vi "GetDataFiles.vi"(4 "Color scheme":string, 6 "Settings":T1={"Name of test"="", "Date"=timestamp(0 s since 1904-01-01), "Location"="", "Template"="", "Soundcard"="", "resolution"=32, "Sampling rate"=48000, "Ch1 Gain "=25.0, "Ch2 Gain"=10.0, "Sample time (s)"=0.3, "Pre-trigger (s)"=0.01, "Hammer Threshold"=10.0, "Positions"=12, "Taps/Position"=5, "Set Names"="", "Freq resolution"=10.0, "Hammer cutoff"=0.0, "Mic cutoff"=0.0, "Double bounce "=0.0, "Hammer Cal"=10.0, "dB Offset"=0.0, "Accel Cal"=10.0, "Vibrometer Cal"=0.0, "Mic Cal"=0.0, "Output"=2, "Voltage Cal"=1.0, "Vibrometer Port"="ASRL27::INSTR", "Range"=4, "High Pass"=2, "Bandwidth"=4, "X Range"=[], "Y Range"=[], "dB Spread"=0.0, "Trigger"=0, "Ch_1"=25, "Ch_2"=25, "flip?"=FALSE, "60Hz"=FALSE, "Time offset"=0.0, "Piezo Cal"=1.0, "Default Notes"=""} {"Ch_2" min=1 step=1; "Ch_1" min=1 max=100 step=1; "Trigger" items=["Hammer (force)", "Self-tap", "Spacebar"]; "Bandwidth" items=["1 kHz"=1, "5 kHz"=5, "10 kHz"=10, "25 kHz"=25, "50 kHz"=50, "100 kHz"=100]; "High Pass" items=["Off", "13 Hz", "104 Hz"]; "Range" items=["10 mm/s"=1, "20 mm/s"=2, "50 mm/s"=5, "100 mm/s"=10, "200 mm/s"=20, "500 mm/s"=50, "1 m/s"=100, "2 m/s"=200]; "Output" items=["Accelerometer", "Speed (from acceleration)", "Microphone", "Vibrometer", "Piezo"]; "Voltage Cal" format="%#_13g"; "Ch2 Gain" format="%#_13g"; "Ch1 Gain" format="%#_13g"; "Double bounce" min=0.0; "Mic cutoff" min=0.0 format="%#_4g"; "Hammer cutoff" min=0.0 format="%#_4g"; "Freq resolution" min=0.0; "Pre-trigger (s)" format="%#_13g"; "Date" format="%<%H:%M\n%d/%m/%y>T"; "resolution" items=["16 bit"=16, "24 bit"=24, "32 bit"=32]; "Sampling rate" items=["22050 samp/s"=22050, "44100 samp/s"=44100, "48000 samp/s"=48000]}, 7 "View":u16(ring) items=["Raw", "Volts", "Units (Pa, N, etc)"], 8 "plots":refnum<vi>[](array[refnum]), 9 "Show history":bool, 10 "path":path, 11 "Method":enum16{"Sqrt(H1H2)", "H1", "H2"}(ring)) -> (0 "Microphone":cluster{dbl, "dt":dbl, "Y":dbl[]}[](graph), 1 "Average FRF":cluster{dbl, "df":dbl, dbl[]}[](graph), 2 "Last Data Set":waveform(dbl)[](array[waveform]), 3 "Hammer":cluster{dbl, "dt":dbl, "Y":dbl[]}[](graph), 5 "Hammer Spectra":cluster{dbl, "df":dbl, "FFT {X}":dbl[]}[](array[cluster]))   [LabVIEW 2022 SP3]
uses:
  PreferencesControl.ctl
  Mic/Mic_Global.vi
panel:
  out "Line":dbl
  out "Banner":string
  # "Hz"
  # "dB"
  # "dB"
  # "sec"
  # "sec"
  # "mV/Pa"
  # "mV/m/s2"
  # "mV/mm/s"
  # "V/N"
  # "sec"
  # "sec"
  # "mV/N"
  # "a.u."
  # "a.u."
  # "sec"
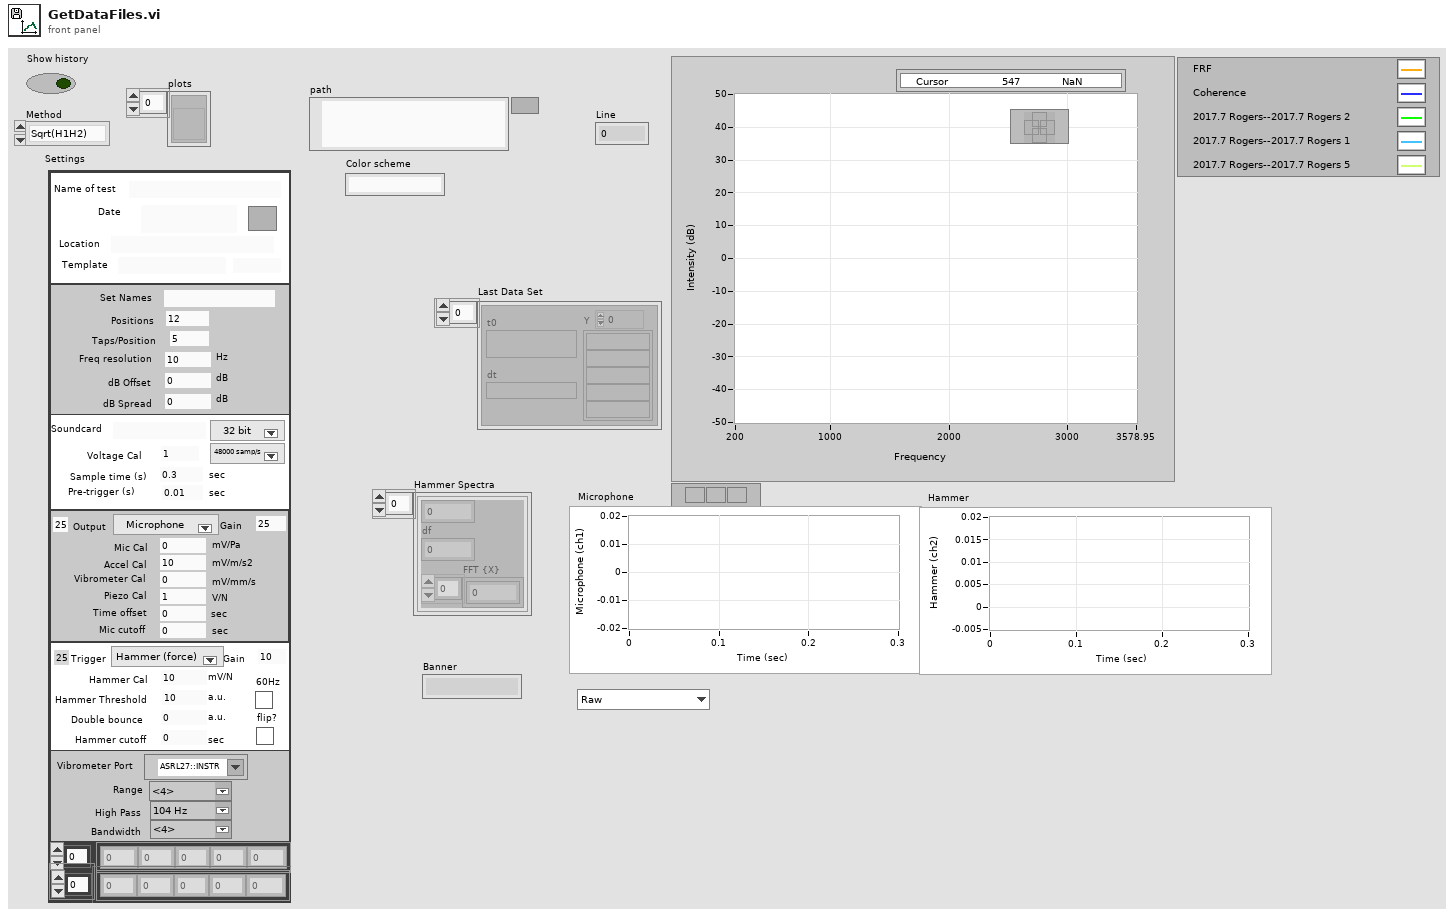
[diagram p1: front panel]
types:
  T1 = typedef "PreferencesControl.ctl" = cluster{"Name of test":string, "Date":timestamp, "Location":string, "Template":string, "Soundcard":string, "resolution":u16, "Sampling rate":u16, "Ch1 Gain ":dbl, "Ch2 Gain":dbl, "Sample time (s)":dbl, "Pre-trigger (s)":dbl, "Hammer Threshold":dbl, "Positions":i16, "Taps/Position":i16, "Set Names":string, "Freq resolution":dbl, "Hammer cutoff":dbl, "Mic cutoff":dbl, "Double bounce ":dbl, "Hammer Cal":dbl, "dB Offset":dbl, "Accel Cal":dbl, "Vibrometer Cal":dbl, "Mic Cal":dbl, "Output":u16, "Voltage Cal":dbl, "Vibrometer Port":refnum<visa-resource-name>, "Range":u16, "High Pass":u16, "Bandwidth":u16, "X Range":cluster{"Minimum":dbl, "Maximum":dbl, "Increment":dbl, "Minor Increment":dbl, "Start":dbl}[], "Y Range":cluster{"Minimum":dbl, "Maximum":dbl, "Increment":dbl, "Minor Increment":dbl, "Start":dbl}[], "dB Spread":dbl, "Trigger":u16, "Ch_1":u8, "Ch_2":u8, "flip?":bool, "60Hz":bool, "Time offset":dbl, "Piezo Cal":dbl, "Default Notes":string}
  T2 = cluster{"Hammer":cluster{dbl, "dt":dbl, "Y":dbl[]}[], "Microphone":cluster{dbl, "dt":dbl, "Y":dbl[]}[], "Hammer Spectrum":cluster{dbl, "dt":dbl, "Y":dbl[]}[], "FRF":cluster{dbl, "dt":dbl, "Y":dbl[]}[]}
  T3 = cluster{"Alerts":bool, "Log X Axis":bool, "dB scale":bool, "Averaging":bool, "Fade":dbl, "Centroids?":bool, "line thickness":u8}
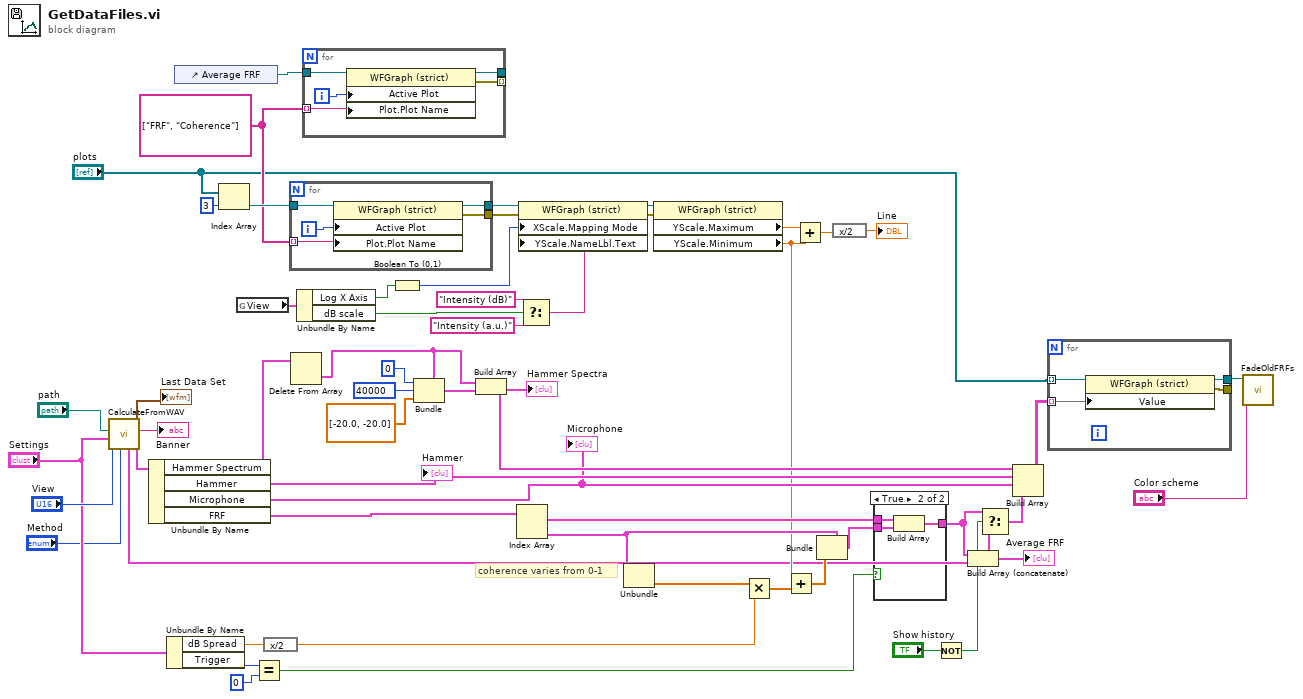
[diagram p0: block diagram]
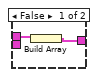
[diagram p2: hidden frame]
diagram:
  w40 = string[] ["FRF", "Coherence"]
  # "coherence varies from 0-1"
  n1 = call "CalculateFromWAV.vi"("Method"="Method", "View"="View", "Settings"="Settings", "path"="path") -> ("Plots"=w44:T2, "Alert"=→"Banner":string, "Last Data Set"=→"Last Data Set":waveform(dbl)[], "Old FRFs"=w10:cluster{dbl, "dt":dbl, "Y":dbl[]}[])  [unwired: 3 in, 1 out]
  n2 = Unbundle By Name(w44) -> ("Hammer Spectrum"=w43:cluster{dbl, "dt":dbl, "Y":dbl[]}[], "Hammer"=w34:cluster{dbl, "dt":dbl, "Y":dbl[]}[], "Microphone"=w33:cluster{dbl, "dt":dbl, "Y":dbl[]}[], "FRF"=w41:cluster{dbl, "dt":dbl, "Y":dbl[]}[])
  "Microphone" <- w33
  "Hammer" <- w34
  n3 = Unbundle By Name("Settings") -> ("dB Spread"=w13:dbl, "Trigger"=w27:u16)
  n4 = control-ref of="Average FRF"() -> (w48:refnum<vi>)
  n5 = Index Array(array="plots", index=3) -> (element=w51:refnum<vi>)
  n6 = global read "Mic_Global.vi" "View"() -> (w45:T3)
  n7 = Equal?(x=w27, y=u16 0 ("Input")) -> (x = y?=w26:bool)
  n8 = expression code="x/2"(w13) -> (w11:dbl)
  n9 = for {
    tunnel: w51 -> [w61]
    tunnel: w40 -> [w60] mode=indexing
    tunnel: [w59] -> w47
    tunnel: [w58] -> w30
    i -> [w62]
    n10 = property on="Property Node" class="WFGraph (strict)"(reference=w61, "Active Plot"=w62, "Plot.Plot Name"=w60) -> (reference out=w59:refnum<vi>, error out=w58:errorcluster)  [unwired: 1 in]
  }
  n11 = Delete From Array(array=w43) -> (deleted portion=w53:cluster{dbl, "dt":dbl, "Y":dbl[]})  [unwired: 2 in, 1 out]
  n12 = Unbundle By Name(w45) -> ("Log X Axis"=w25:bool, "dB scale"=w21:bool)
  n13 = for {
    tunnel: w48 -> [w66]
    tunnel: [w65] -> _
    tunnel: [w64] -> _ mode=indexing
    tunnel: w40 -> [w63] mode=indexing
    i -> [w67]
    n14 = property on="Property Node" class="WFGraph (strict)"(reference=w66, "Active Plot"=w67, "Plot.Plot Name"=w63) -> (reference out=w65:refnum<vi>, error out=w64:errorcluster)  [unwired: 1 in]
  }
  n15 = Boolean To (0,1)(Boolean=w25) -> (0, 1=w46:i16)
  n16 = Bundle(cluster=w53, 0, "dt"=40000, "Y"=dbl[] [-20.0, -20.0]) -> (w57:cluster{dbl, "dt":dbl, "Y":dbl[]})
  n17 = Build Array(w53, w57) -> (w35:cluster{dbl, "dt":dbl, "Y":dbl[]}[])
  "Hammer Spectra" <- w35
  n18 = Index Array(array=w41) -> (element #1=w36:cluster{dbl, "dt":dbl, "Y":dbl[]}, element #2=w42:cluster{dbl, "dt":dbl, "Y":dbl[]})  [unwired: 2 in]
  n19 = Select(t="Intensity (dB)" ("Position"), s=w21, f="Intensity (a.u.)" ("Position")) -> (s? t:f=w22:string)
  n20 = property on="Property Node" class="WFGraph (strict)"(reference=w47, error in=w30, "XScale.Mapping Mode"=w46, "YScale.NameLbl.Text"=w22) -> (reference out=w20:refnum<vi>, error out=w4:errorcluster)
  n21 = Unbundle(w42) -> ("Y"=w12:dbl[])  [unwired: 2 out]
  n22 = property on="Property Node" class="WFGraph (strict)"(reference=w20, error in=w4) -> ("YScale.Maximum"=w19:dbl, "YScale.Minimum"=w17:dbl)  [unwired: 2 out]
  n23 = Multiply(x=w12, y=w11) -> (x*y=w14:dbl[])
  n24 = Add(x=w17, y=w14) -> (x+y=w16:dbl[])
  n25 = Add(x=w19, y=w17) -> (x+y=w18:dbl)
  n26 = Bundle(cluster=w42, "Y"=w16) -> (w38:cluster{dbl, "dt":dbl, "Y":dbl[]})  [unwired: 2 in]
  n27 = expression code="x/2"(w18) -> (→"Line":dbl)
  n28 = case shown="True" w26 {
    tunnel: w38 -> [_ w72]
    tunnel: [w68 w71] -> w7
    tunnel: w36 -> [w69 w70]
    frame False {
      n29 = Build Array(w69) -> (w68:cluster{dbl, "dt":dbl, "Y":dbl[]}[])
    }
    frame True {
      n30 = Build Array(w70, w72) -> (w71:cluster{dbl, "dt":dbl, "Y":dbl[]}[])
    }
  }
  n31 = Not(x="Show history") -> (.not. x?=w5:bool)
  n32 = Build Array (concatenate)(w7, w10) -> (w2:cluster{dbl, "dt":dbl, "Y":dbl[]}[])
  "Average FRF" <- w2
  n33 = Select(t=w7, s=w5, f=w2) -> (s? t:f=w6:cluster{dbl, "dt":dbl, "Y":dbl[]}[])
  n34 = Build Array(w35, w34, w33, w6) -> (w37:cluster{dbl, "dt":dbl, "Y":dbl[]}[][])
  n35 = for {
    tunnel: "plots" -> [w76] mode=indexing
    tunnel: w37 -> [w74] mode=indexing
    tunnel: [w75] -> _
    tunnel: [w73] -> w3
    n36 = property on="Property Node" class="WFGraph (strict)"(reference=w76, "Value"=w74) -> (reference out=w73:refnum<vi>, error out=w75:errorcluster)  [unwired: 1 in]
  }
  n37 = call "FadeOldFRFs.vi"("Color scheme"="Color scheme", "WaveformGraph in"=w3) -> ()  [unwired: 10 in]
